vi "Tosca-Analog Output Thread (new).vi"(0 "Tosca Output Queue":refnum<queue>, 2 "IPC":T1, 7 "pts/frame":i32=10, 11 "Fs (Hz)":dbl) -> (15 "error out":errorcluster)   [LabVIEW 2020]
uses:
  Typedefs/Tosca-State AODO.ctl
  Typedefs/Tosca-AO Runtime.ctl
  Typedefs/Tosca-DO Runtime.ctl
  epl-vi-lib/Signal Synthesis VIs/4th Generation/Classes/SignalManager/SignalManager.lvclass
  IPC VIs/Tosca-IPC.ctl
  Classes/Parameters/Parameters.lvclass
  Digital Input VIs/Tosca-DI Queue Data.ctl
  Digital Input VIs/Tosca-Input Event.ctl
  Digital Input VIs/Tosca-Input Criterion.ctl
  epl-vi-lib/Utility VIs/Type Defs/Logic State.ctl
  Typedefs/Tosca-Accumulator.ctl
  Typedefs/Tosca-Synapse Start Data.ctl
  IPC VIs/Tosca-Message.ctl
  IPC VIs/Tosca-Message Action.ctl
  Typedefs/Tosca-Thread Type.ctl
  Imaging VIs/Tosca-2P-Notifier Data.ctl
  Typedefs/Tosca-MATLAB Queue Data.ctl
  Visual Stim VIs/Tosca-Grating.ctl
  Visual Stim VIs/Tosca-Grating Type.ctl
  Typedefs/Tosca-File IO Notification.ctl
  Typedefs/Tosca-AODO Data.ctl
  Trace VIs/Tosca-Trace-Event.ctl
  Tosca-Globals.vi
panel:
  out "Parser error":errorcluster
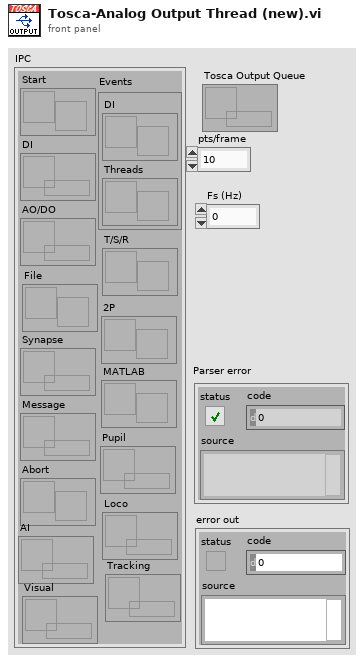
[diagram p1: front panel]
types:
  T1 = typedef "Tosca-IPC.ctl" = cluster{"Start":refnum<notifier>, "DI":refnum<queue>, "AO/DO":refnum<queue>, "Synapse":refnum<queue>, "Message":refnum<queue>, "Abort":refnum<notifier>, "Events":cluster{"DI":refnum<user-event>, "Threads ":refnum<user-event>}, "T/S/R":refnum<notifier>, "2P":refnum<notifier>, "MATLAB":refnum<notifier>, "Pupil":refnum<queue>, "Loco":refnum<queue>, "AI":refnum<queue>, "Tracking":refnum<queue>, "Visual":refnum<queue>, "File":refnum<notifier>}
  T2 = typedef "Tosca-Trace-Event.ctl" = enum16{"Unspecified", "Trial start", "Enqueue", "Result", "End parser", "Frame", "Queue available", "Timeout sent", "WritePos", "TTL"}
  T3 = typedef "Tosca-AODO Data.ctl" = cluster{"AO":dbl[][], "DO":bool[][], "frame":i32, "stop":bool}
  T4 = typedef "Tosca-Thread Type.ctl" = enum16{"None", "AODO", "Masker", "ET", "Imaging", "Pupil", "AI", "DI", "Camera", "TTL out", "Loco", "Visual"}
  T5 = typedef "Tosca-State AODO.ctl" = cluster{"Name":string, "T (s)":dbl, "First AO":dbl[][], "frames/rep":i32, "finish?":bool, "Nrep":i32, "AO":T6, "DO":T7, "immediate":bool, "First DO":bool[][], "SigMan":refnum<class "SignalManager.lvclass">}
  T6 = typedef "Tosca-AO Runtime.ctl" = cluster{"Fs (Hz)":dbl, "pts/frame":i32, "pts/rep":i32, "ramp off":bool[], "fade out":dbl[][]}
  T7 = typedef "Tosca-DO Runtime.ctl" = cluster{"Fs (Hz)":dbl, "pts/frame":i32, "pts/rep":i32, "Rep":i32, "State":i32, "Trial":i32, "Frame":i32, "frOut":bool[], "Nchan":i32}
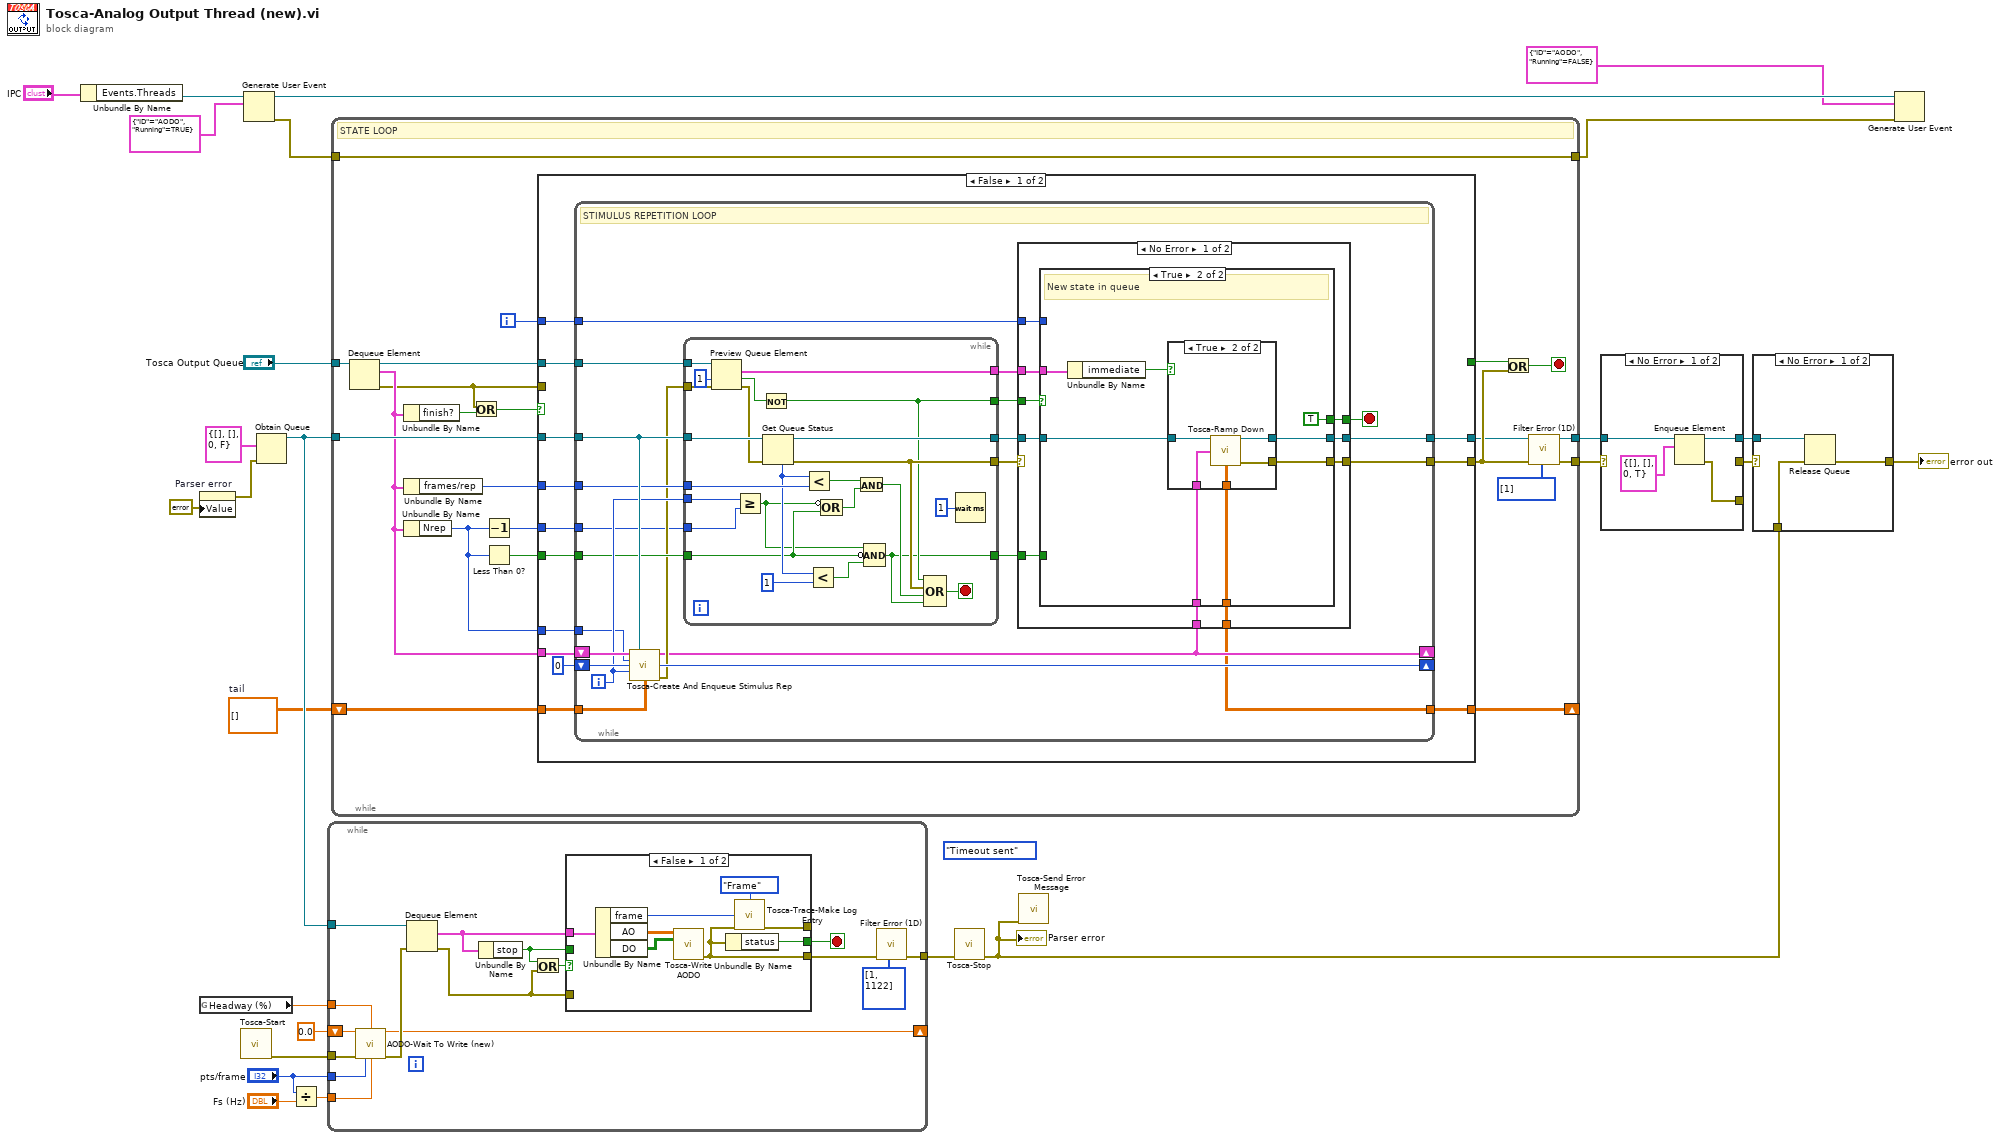
[diagram p0: block diagram]
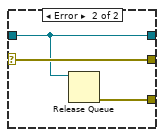
[diagram p3: hidden frame]
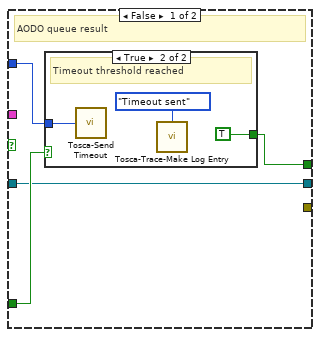
[diagram p4: hidden frame]
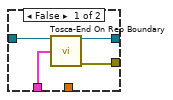
[diagram p6: hidden frame]
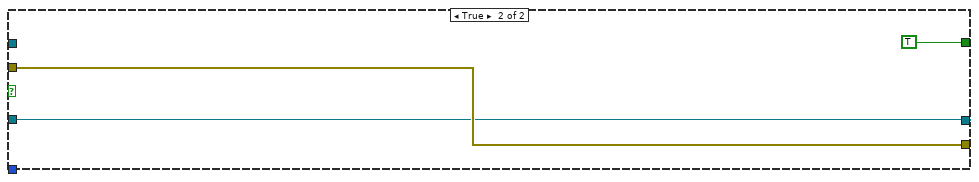
[diagram p8: hidden frame]
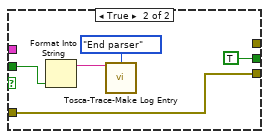
[diagram p9: hidden frame]
diagram:
  w1 = dbl[][] []  # tail
  (unwired) Tosca-Trace-Event."Timeout sent" ("Event")
  n1 = Unbundle By Name("IPC") -> ("Events.Threads"=w24:refnum<user-event>)
  n2 = property on="Parser error" class="Clust (strict)"("Value"=errorcluster {"status"=FALSE, "code"=0, "source"=""} ("Parser error")) -> (error out=w14:errorcluster)  [unwired: 2 in, 1 out]
  n3 = global read "Tosca-Globals.vi" "Headway (%)"() -> (w5:dbl)
  n4 = call "Tosca-Start.vi"() -> ("error out"=w7:errorcluster)  [unwired: 15 in]
  n5 = Generate User Event(user event=w24, event data cluster=cluster{"ID":T4, "Running":bool} {"ID"=enum."AODO", "Running"=TRUE} ("event data")) -> (user event out=w22:refnum<user-event>, error out=w15:errorcluster)  [unwired: 2 in]
  n6 = Obtain Queue(element data type=T3 {"AO"=[], "DO"=[], "frame"=0, "stop"=FALSE}, error in (no error)=w14) -> (queue out=w18:refnum<queue>)  [unwired: 3 in, 2 out]
  n7 = Divide(x="pts/frame", y="Fs (Hz)") -> (x/y=w2:dbl)
  n8 = while {
    tunnel: w18 -> [w42]
    tunnel: w7 -> [w33]
    tunnel: [w39] -> w19
    shift-right: [w30] -> _
    shift-left: 0.0 -> [w32]
    tunnel: w5 -> [w29]
    tunnel: "pts/frame" -> [w28]
    tunnel: w2 -> [w27]
    stop <- w35 stop-if-true
    n9 = call "AODO-Wait To Write (new).vi"("Tnext in"=w32, "Headway"=w29, "error in (no error)"=w33, "Frame size"=w28, "Poll (s)"=w27) -> ("Tnext out"=w30:dbl, "error out"=w31:errorcluster)  [unwired: 9 in]
    n10 = Dequeue Element(queue=w42, error in (no error)=w31) -> (element=w38:T3, error out=w36:errorcluster)  [unwired: 1 in, 2 out]
    n11 = Unbundle By Name(w38) -> ("stop"=w34:bool)
    n12 = Or(x=w34, y=w36) -> (x .or. y?=w37:bool)
    n13 = case shown="False" w37 {
      tunnel: w38 -> [w50 _]
      tunnel: [w45 w55] -> w40
      tunnel: [w47 _] -> _
      tunnel: w36 -> [_ w55]
      tunnel: [w46 TRUE ("status")] -> w35
      tunnel: w34 -> [_ w51]
      frame False {
        n14 = Unbundle By Name(w50) -> ("frame"=w43:i32, "AO"=w49:dbl[][], "DO"=w44:bool[][])
        n15 = call "Tosca-Write AODO.vi"("AO"=w49, "DO"=w44) -> ("error out"=w45:errorcluster)  [unwired: 13 in]
        n16 = Unbundle By Name(w45) -> ("status"=w46:bool)
        n17 = call "Tosca-Trace-Make Log Entry.vi"("Event"=Tosca-Trace-Event."Frame", "Value"=w43, "error in (no error)"=w45) -> ("error out"=w47:errorcluster)  [unwired: 12 in]
      }
      frame True {
        n18 = Format Into String(w51) -> (resulting string=w52:string)  [unwired: 3 in, 1 out]
        n19 = call "Tosca-Trace-Make Log Entry.vi"("Message"=w52, "Event"=Tosca-Trace-Event."End parser") -> ()  [unwired: 13 in, 1 out]
      }
    }
    n20 = call "Filter Error (1D).vi"("error in (no error)"=w40, "Array"=i32[] [1, 1122]) -> ("error out"=w39:errorcluster)  [unwired: 9 in]
  }
  n21 = while {
    tunnel: "Tosca Output Queue" -> [w76]
    tunnel: w18 -> [w74]
    tunnel: [w67] -> w13
    tunnel: [w66] -> w16
    tunnel: w15 -> [w66]
    tunnel: [w65] -> w12
    shift-right: [w57] -> _
    shift-left: w1 -> [w58]
    i -> [w71]
    stop <- w70 stop-if-true
    # "STATE LOOP"
    n22 = Dequeue Element(queue=w76) -> (queue out=w75:refnum<queue>, element=w64:T5, error out=w62:errorcluster)  [unwired: 2 in, 1 out]
    n23 = Unbundle By Name(w64) -> ("finish?"=w63:bool)
    n24 = Unbundle By Name(w64) -> ("frames/rep"=w73:i32)
    n25 = Unbundle By Name(w64) -> ("Nrep"=w56:i32)
    n26 = Or(x=w62, y=w63) -> (x .or. y?=w61:bool)
    n27 = Decrement(x=w56) -> (x-1=w59:i32)
    n28 = Less Than 0?(x=w56) -> (x < 0?=w60:bool)
    n29 = case shown="False" w61 {
      tunnel: w75 -> [w89 _]
      tunnel: w74 -> [w87 w173]
      tunnel: w73 -> [w86 _]
      tunnel: w64 -> [w85 _]
      tunnel: [w83 w175] -> w68
      tunnel: [_ TRUE] -> w72
      tunnel: w71 -> [w84 _]
      tunnel: [w82 w173] -> w65
      tunnel: w60 -> [w81 _]
      tunnel: w62 -> [_ w175]
      tunnel: w59 -> [w80 _]
      tunnel: w58 -> [w79 _]
      tunnel: [w78 _] -> w57
      tunnel: w56 -> [w77 _]
      frame False {
        n30 = while {
          tunnel: w89 -> [w109]
          shift-right: [w94] -> _
          shift-left: w85 -> [w112]
          shift-right: [w110] -> _
          shift-left: 0 -> [w111]
          tunnel: w87 -> [w108]
          tunnel: w86 -> [w107]
          tunnel: w84 -> [w100]
          tunnel: [w99] -> w83
          tunnel: [w97] -> w82
          tunnel: w81 -> [w96]
          tunnel: w80 -> [w93]
          tunnel: w79 -> [w92]
          tunnel: [w91] -> w78
          tunnel: w77 -> [w90]
          i -> [w98]
          stop <- w101 stop-if-true
          # "STIMULUS REPETITION LOOP"
          n31 = call "Tosca-Create And Enqueue Stimulus Rep.vi"("Stim data in"=w112, "AODO Queue"=w108, "Nreps"=w90, "Nqueue in"=w111, "Rep"=w98, "tail"=w92) -> ("Stim data out"=w94:T5, "Nqueue out"=w110:i32, "error out"=w95:errorcluster)  [unwired: 7 in]
          n32 = while {
            tunnel: w109 -> [w172]
            tunnel: w108 -> [w171]
            tunnel: w107 -> [w170]
            tunnel: [w168] -> w102
            tunnel: [w160] -> w105
            tunnel: [w155] -> w104
            tunnel: [w162] -> w106
            tunnel: [w158] -> w103
            tunnel: w98 -> [w157]
            tunnel: w96 -> [w151]
            tunnel: w95 -> [w154]
            tunnel: w93 -> [w152]
            stop <- w163 stop-if-true
            n33 = Preview Queue Element(queue=w172, timeout in ms (-1)=1, error in (no error)=w154) -> (element=w158:T5, timed out?=w161:bool, error out=w166:errorcluster)  [unwired: 1 out]
            n34 = Greater Or Equal?(x=w157, y=w152) -> (x >= y?=w149:bool)
            n35 = Not(x=w161) -> (.not. x?=w160:bool)
            n36 = Get Queue Status(queue=w171, error in (no error)=w166) -> (queue out=w168:refnum<queue>, error out=w162:errorcluster, # elements in queue=w169:i32)  [unwired: 1 in, 5 out]
            n37 = Less?(x=w169, y=w170) -> (x < y?=w165:bool)
            n38 = Less?(x=w169, y=1) -> (x < y?=w164:bool)
            n39 = Compound Arithmetic op=OR(invert w149, w151) -> (w150:bool)
            n40 = And(x=w165, y=w150) -> (x .and. y?=w156:bool)
            n41 = Compound Arithmetic op=AND(w149, invert w151, w164) -> (w155:bool)
            n42 = Compound Arithmetic op=OR(w160, w162, w156, w155) -> (w163:bool)
            n43 = Wait (ms)(milliseconds to wait=u32 1) -> ()  [unwired: 1 out]
          }
          n44 = case shown="No Error" w106 {
            selector: w106 -> [_ w148]
            tunnel: w105 -> [w122 _]
            tunnel: w104 -> [w121 _]
            tunnel: w103 -> [w120 _]
            tunnel: w102 -> [w119 w147]
            tunnel: [w118 _] -> w101
            tunnel: w100 -> [w117 _]
            tunnel: [w115 w148] -> w99
            tunnel: [w116 w147] -> w97
            tunnel: w94 -> [w114 _]
            tunnel: [w113 _] -> w91
            frame No Error {
              n45 = case shown="True" w122 {
                tunnel: w121 -> [w124 _]
                tunnel: w120 -> [_ w137]
                tunnel: w119 -> [w123 w135]
                tunnel: [w125 TRUE] -> w118
                tunnel: w117 -> [w126 _]
                tunnel: [w123 w134] -> w116
                tunnel: [_ w133] -> w115
                tunnel: w114 -> [_ w131]
                tunnel: [_ w130] -> w113
                frame False {
                  # "AODO queue result"
                  n46 = case shown="True" w124 {
                    tunnel: w126 -> [_ w128]
                    tunnel: [_ TRUE] -> w125
                    frame False {
                      # "Create and enqueue new stimulus rep"
                    }
                    frame True {
                      # "Timeout threshold reached"
                      n47 = call "Tosca-Send Timeout.vi"("State"=w128) -> ()  [unwired: 15 in]
                      n48 = call "Tosca-Trace-Make Log Entry.vi"("Event"=Tosca-Trace-Event."Timeout sent") -> ()  [unwired: 14 in, 1 out]
                    }
                  }
                }
                frame True {
                  # "New state in queue"
                  n49 = Unbundle By Name(w137) -> ("immediate"=w132:bool)
                  n50 = case shown="True" w132 {
                    tunnel: w135 -> [w141 w146]
                    tunnel: [w140 w145] -> w134
                    tunnel: [w138 w144] -> w133
                    tunnel: w131 -> [w139 w143]
                    tunnel: [_ w142] -> w130
                    frame False {
                      n51 = call "Tosca-End On Rep Boundary.vi"("Queue in"=w141, "Stim data in"=w139) -> ("Queue out"=w140:refnum<queue>, "error out"=w138:errorcluster)  [unwired: 12 in]
                    }
                    frame True {
                      n52 = call "Tosca-Ramp Down.vi"("Queue in"=w146, "Stim data in"=w143) -> ("Queue out"=w145:refnum<queue>, "tail"=w142:dbl[][], "error out"=w144:errorcluster)  [unwired: 11 in]
                    }
                  }
                }
              }
            }
            frame Error {
            }
          }
        }
      }
      frame True {
      }
    }
    n53 = Or(x=w72, y=w68) -> (x .or. y?=w70:bool)
    n54 = call "Filter Error (1D).vi"("error in (no error)"=w68, "Array"=i32[] [1]) -> ("error out"=w67:errorcluster)  [unwired: 9 in]
  }
  n55 = call "Tosca-Stop.vi"("error in (no error)"=w19) -> ("error out"=w11:errorcluster)  [unwired: 14 in]
  "Parser error" <- w11
  n56 = call "Tosca-Send Error Message.vi"("error in (no error)"=w11) -> ()  [unwired: 15 in]
  n57 = case shown="No Error" w13 {
    selector: w13 -> [_ w182]
    tunnel: w12 -> [w179 w180]
    tunnel: [_ w182] -> w9
    tunnel: [w176 w181] -> _
    tunnel: [w177 w180] -> w10
    frame No Error {
      n58 = Enqueue Element(queue=w179, element=T3 {"AO"=[], "DO"=[], "frame"=0, "stop"=TRUE}) -> (queue out=w177:refnum<queue>, error out=w176:errorcluster)  [unwired: 2 in, 1 out]
    }
    frame Error {
      n59 = Release Queue(queue=w180) -> (error out=w181:errorcluster)  [unwired: 2 in, 2 out]
    }
  }
  n60 = case shown="No Error" w9 {
    selector: w9 -> [_ w186]
    tunnel: w11 -> [w185 _]
    tunnel: w10 -> [w184 _]
    tunnel: [w183 w186] -> w8
    frame No Error {
      n61 = Release Queue(queue=w184, error in (no error)=w185) -> (error out=w183:errorcluster)  [unwired: 1 in, 2 out]
    }
    frame Error {
    }
  }
  "error out" <- w8
  n62 = Generate User Event(user event=w22, event data cluster=cluster{"ID":T4, "Running":bool} {"ID"=enum."AODO", "Running"=FALSE} ("event data"), error in=w16) -> ()  [unwired: 1 in, 2 out]
